vi "LD.vi"() -> ()   [LabVIEW 2022 SP3]
uses:
  <vilib>/Analysis/baseanly.llb/Mean (DBL).vi
  C:/Users/Public/OneDrive/Desktop/PMT program/SampleCodeLabView/Kinesis_with_LabVIEW_Examples_LV12 - v3/ThorLabs.MotionControl.KCube.DCServoCLI.dll
  PMT program/SampleCodeLabView/Kinesis_with_LabVIEW_Examples_LV12 - v3/ThorLabs.MotionControl.KCube.DCServoCLI.dll
  <vilib>/Utility/file.llb/Write Delimited Spreadsheet (string).vi
  <vilib>/Utility/file.llb/Write Delimited Spreadsheet (DBL).vi
  C:/Users/Public/OneDrive/Desktop/PMT program/SampleCodeLabView/Kinesis_with_LabVIEW_Examples_LV12 - v3/Thorlabs.MotionControl.Controls.dll
  PMT program/SampleCodeLabView/Kinesis_with_LabVIEW_Examples_LV12 - v3/Thorlabs.MotionControl.Controls.dll
  <vilib>/Analysis/NI_AALBase.lvlib
panel:
  in  "Waiting Time for motor":dbl=1500.0
  in  "OE1022D":refnum<visa-resource-name>
  in  "Total Steps":i32
  out "R Phase (B)":dbl[](graph)
  out "R (B)":dbl[](graph)
  out "R Phase (A)":dbl[](graph)
  out "R (A)":dbl[](graph)
  out "AUX-ADC4 (V)":sgl format="%.3f"
  out "AUX-ADC3 (V)":sgl format="%.3f"
  out "AUX-ADC1 (V)":sgl format="%.3f"
  out "AUX-ADC2 (V)":sgl format="%.3f"
  out "R":sgl caption="R (Vrms)" format="%.3p"
  out "X":sgl caption="X (Vrms)" format="%.3p"
  out "Y":sgl caption="Y (Vrms)" format="%.3p"
  out "θ (°)":sgl caption="θ (deg)" format="%.2f"
  out "频率 (Hz)":sgl caption="Freq (Hz)" format="%#.3f"
  out "噪声":sgl caption="Noise(Vrms)" format="%.3p"
  out "Rh1":sgl caption="Rh1 (Vrms)" format="%.3p"
  out "θh1 (°)":sgl caption="θh1 (deg)" format="%.2f"
  out "Rh2":sgl caption="Rh2 (Vrms)" format="%.3p"
  out "Xh2":sgl caption="Xh2 (Vrms)" format="%.3p"
  out "Yh2":sgl caption="Yh2 (Vrms)" format="%.3p"
  out "θh2 (°)":sgl caption="θh2 (deg)" format="%.2f"
  out "Xh1":sgl caption="Xh1 (Vrms)" format="%.3p"
  out "Yh1":sgl caption="Yh1 (Vrms)" format="%.3p"
  out "X 2":sgl caption="X (Vrms)" format="%.3p"
  out "θh2 (°) 2":sgl caption="θh2 (deg)" format="%.2f"
  out "Y 2":sgl caption="Y (Vrms)" format="%.3p"
  out "R 2":sgl caption="R (Vrms)" format="%.3p"
  out "θ (°) 2":sgl caption="θ (deg)" format="%.2f"
  out "频率 (Hz) 2":sgl caption="Freq (Hz)" format="%#.3f"
  out "噪声 2":sgl caption="Noise(Vrms)" format="%.3p"
  out "Rh2 2":sgl caption="Rh2 (Vrms)" format="%.3p"
  out "Yh2 2":sgl caption="Yh2 (Vrms)" format="%.3p"
  out "Xh2 2":sgl caption="Xh2 (Vrms)" format="%.3p"
  out "Xh1 2":sgl caption="Xh1 (Vrms)" format="%.3p"
  out "Yh1 2":sgl caption="Yh1 (Vrms)" format="%.3p"
  out "Rh1 2":sgl caption="Rh1 (Vrms)" format="%.3p"
  out "θh1 (°) 2":sgl caption="θh1 (deg)" format="%.2f"
  in  "file path (dialog if empty) 2":path=path "D:/LabData/Fan Fei/223.txt"
  in  "Lock  in Average Time":i32=500
  in  "Start":dbl
  out "Current Position":dbl
  in  "stepSize":dbl
  in  "direction":i32(ring)=1 items=["Forward"=1, "Backward"=2]
  in  "Motor Controller\nSerialNumber":string="27261255"
  in  "KCubeDCServoControl":refnum<k24>(container)
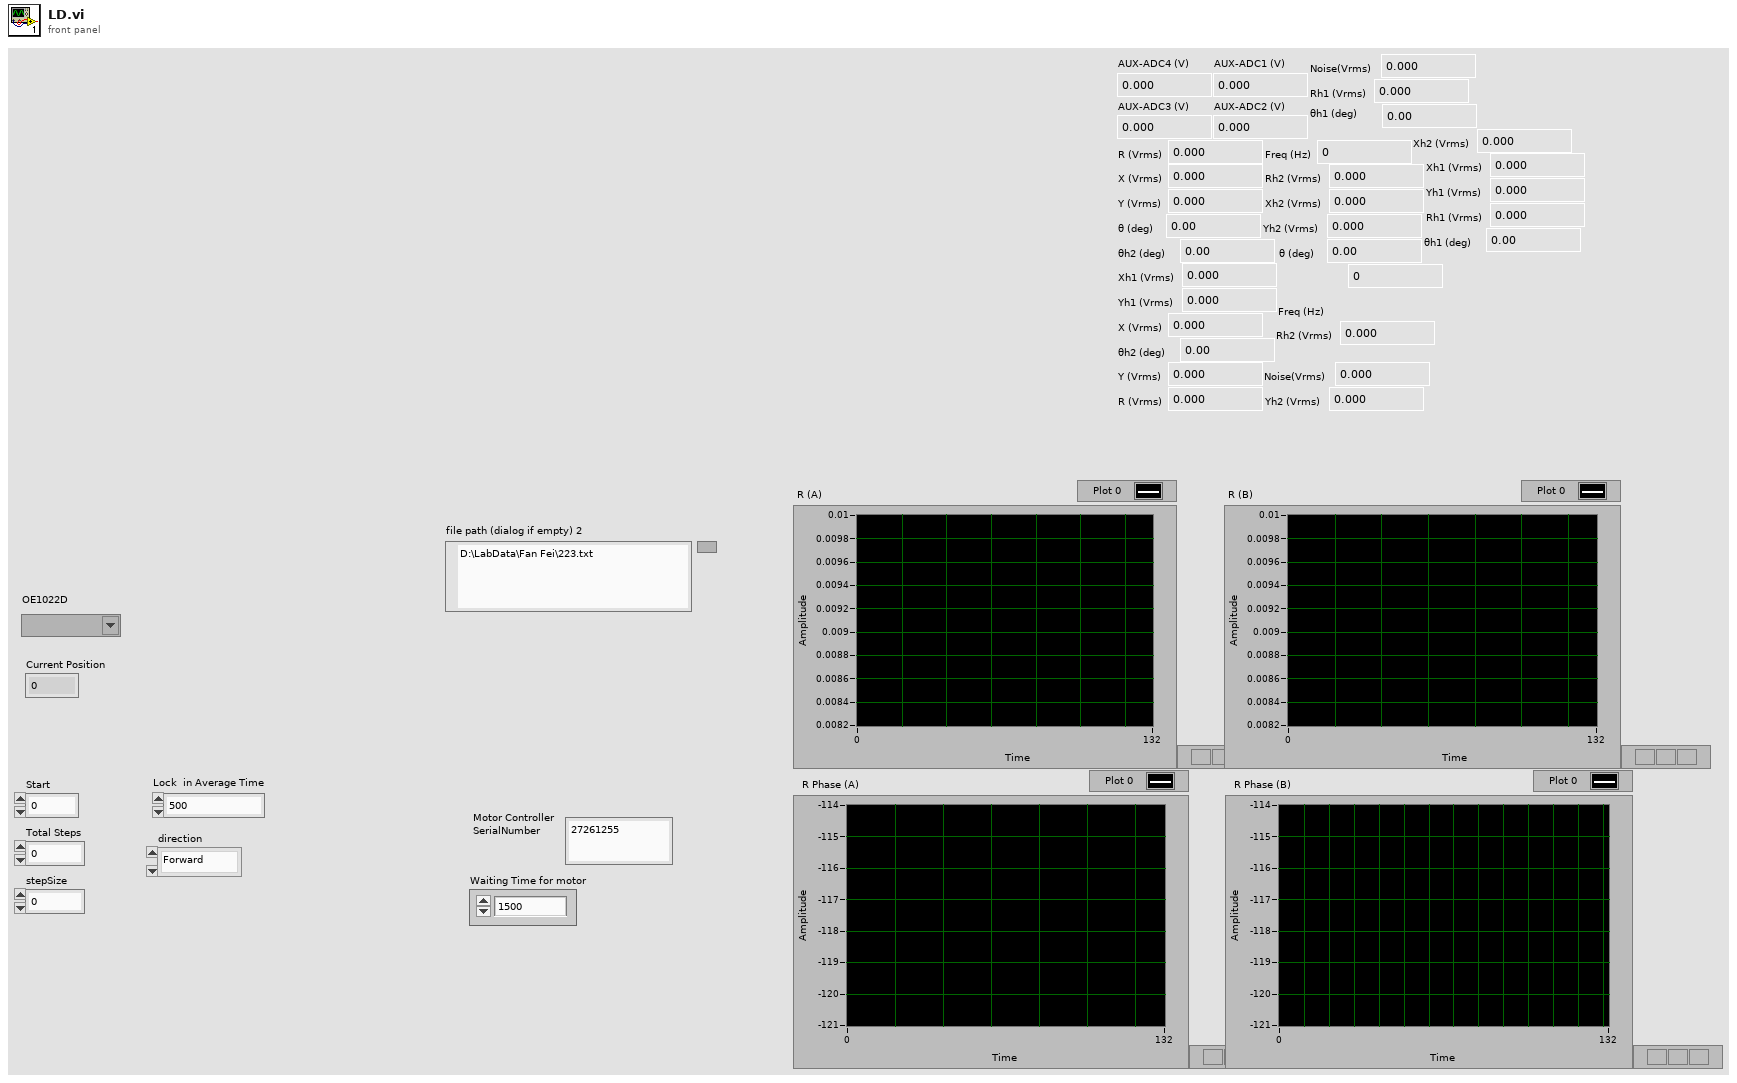
[diagram p1: front panel]
types:
  T1 = cluster{"AD1":dbl[], "AD2":dbl[], "AD3":dbl[], "AD4":dbl[]}
  T2 = cluster{"XB":dbl[], "YB":dbl[], "FrequencyB":dbl[], "NoiseB":dbl[], "Xh1B":dbl[], "Yh1B":dbl[], "Xh2B":dbl[], "Yh2B":dbl[], "Xh2B":dbl[]}
  T3 = cluster{"XA":dbl[], "YA":dbl[], "FrequencyA":dbl[], "NoiseA":dbl[], "Xh1A":dbl[], "Yh1A":dbl[], "Xh2A":dbl[], "Yh2A":dbl[]}
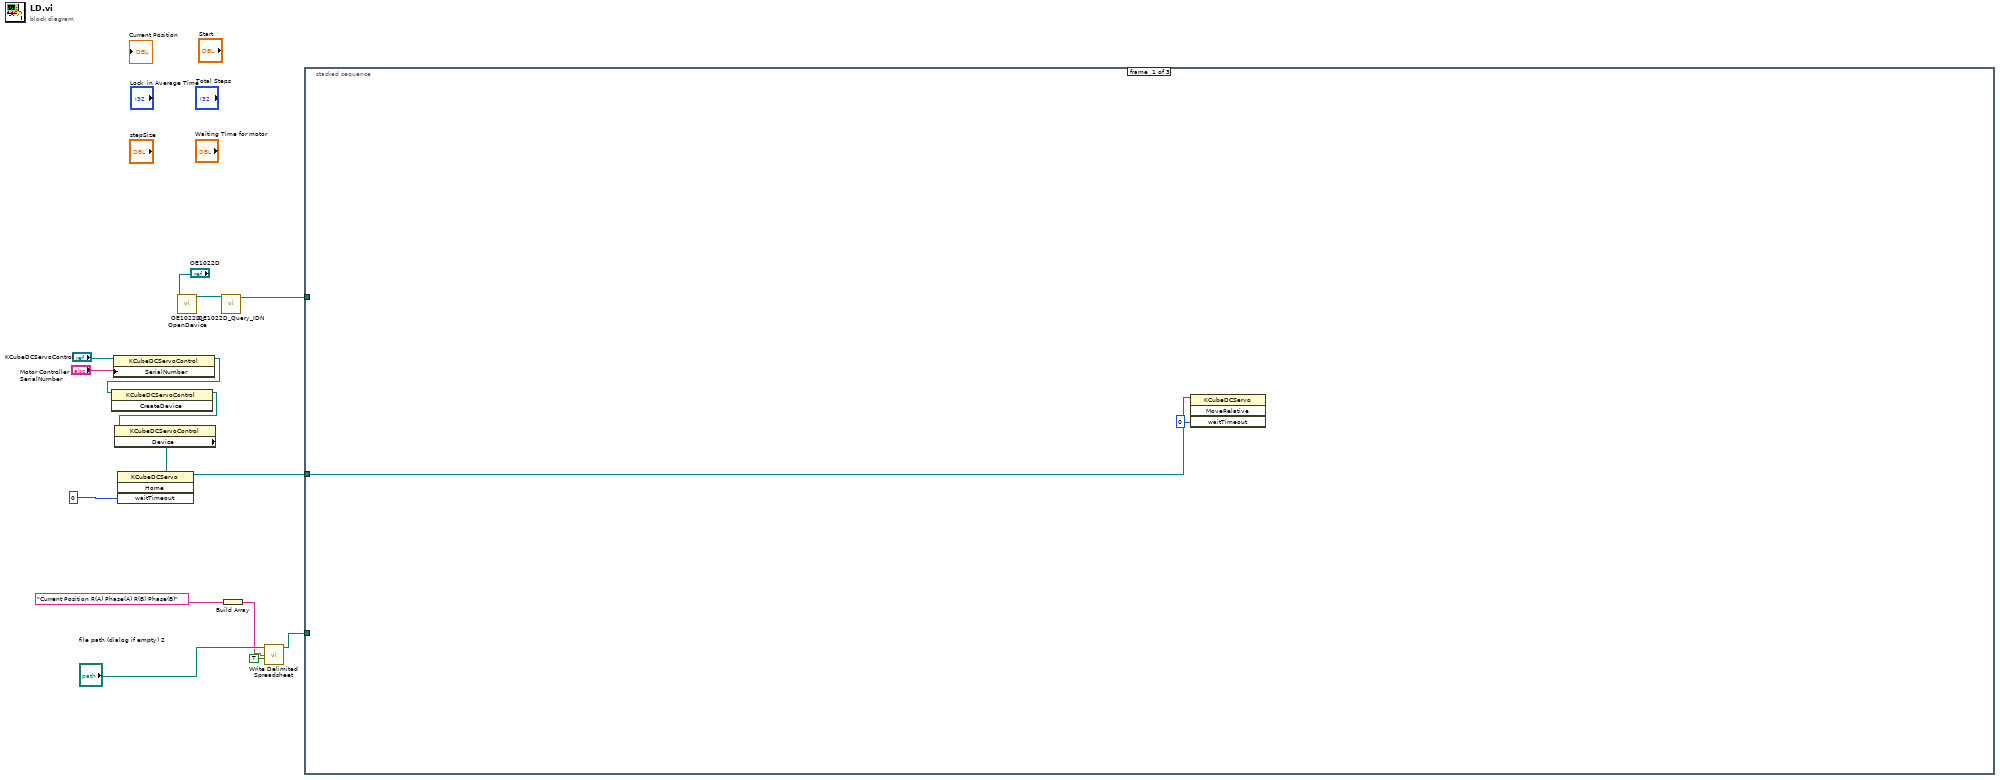
[diagram p0: block diagram]
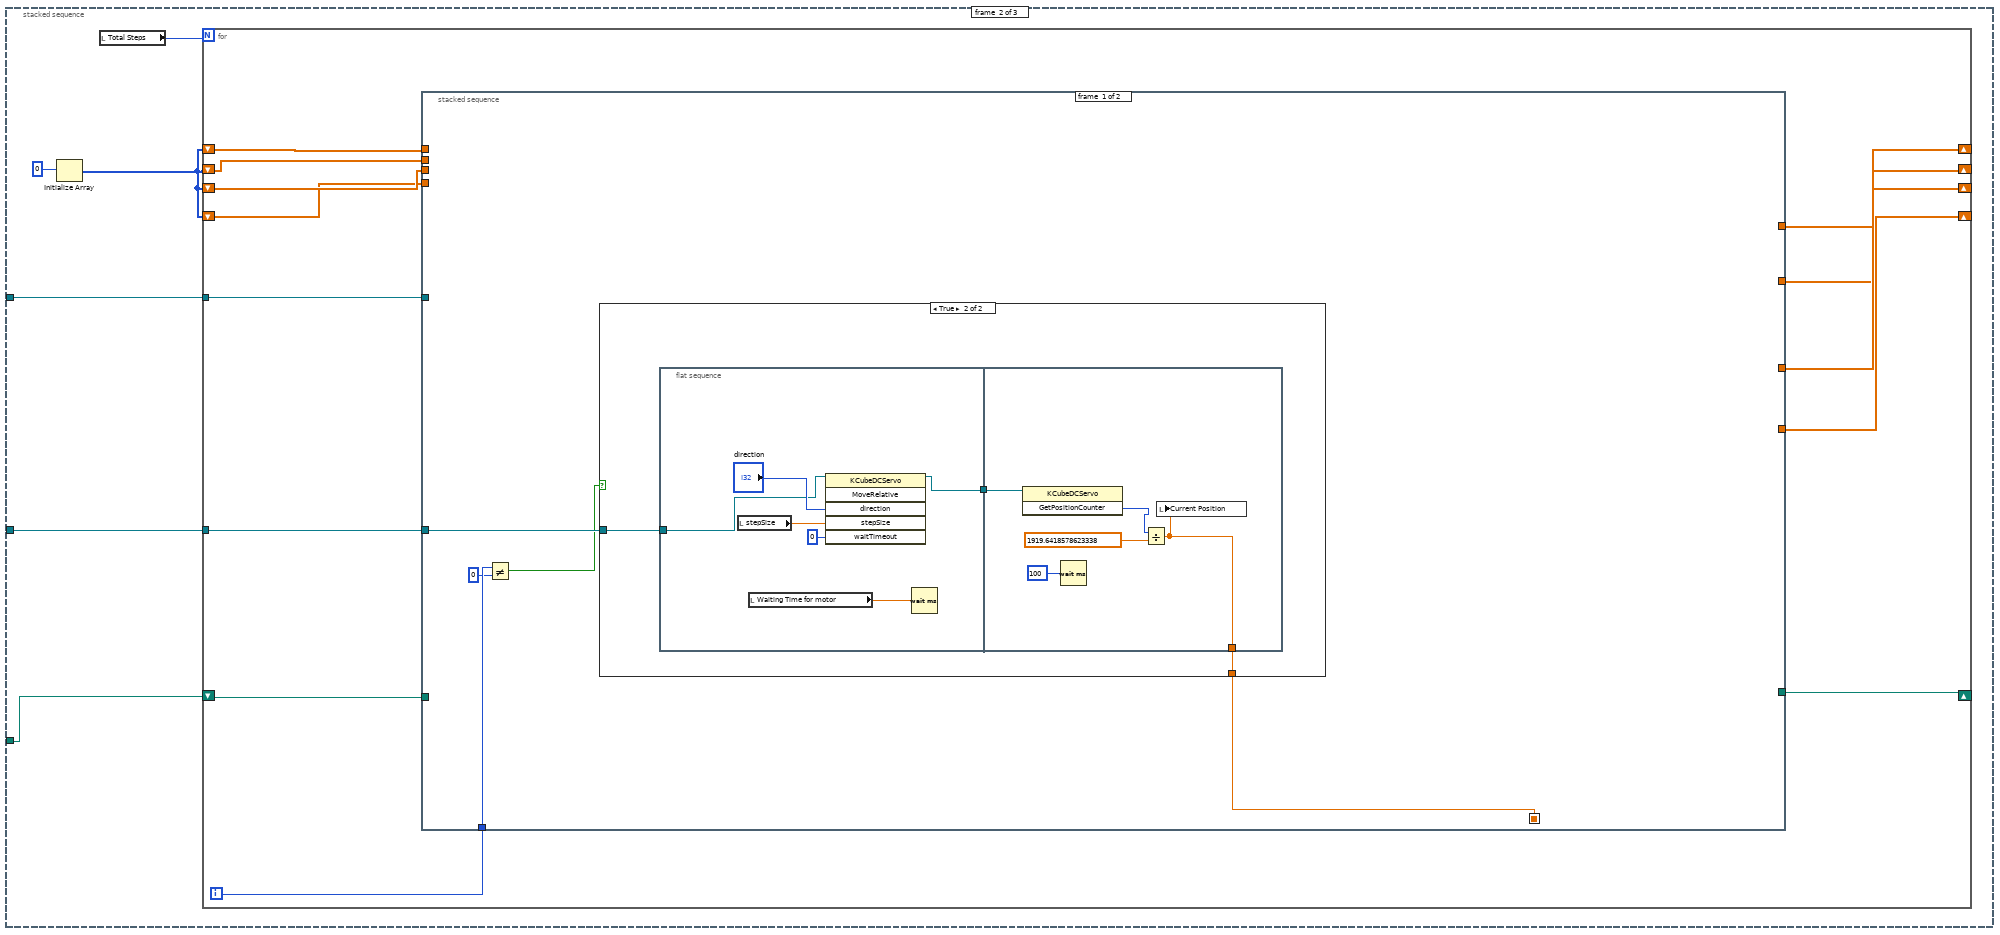
[diagram p2: hidden frame]
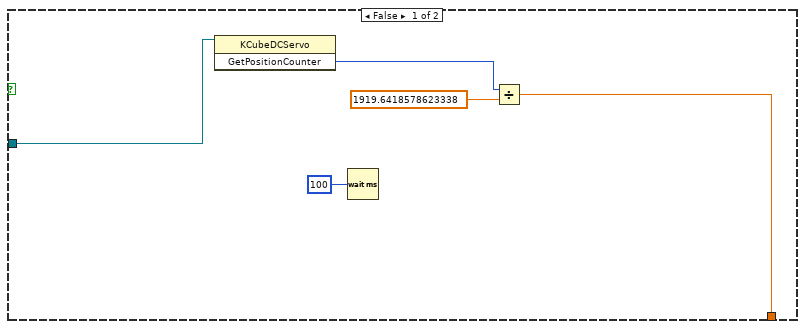
[diagram p3: hidden frame]
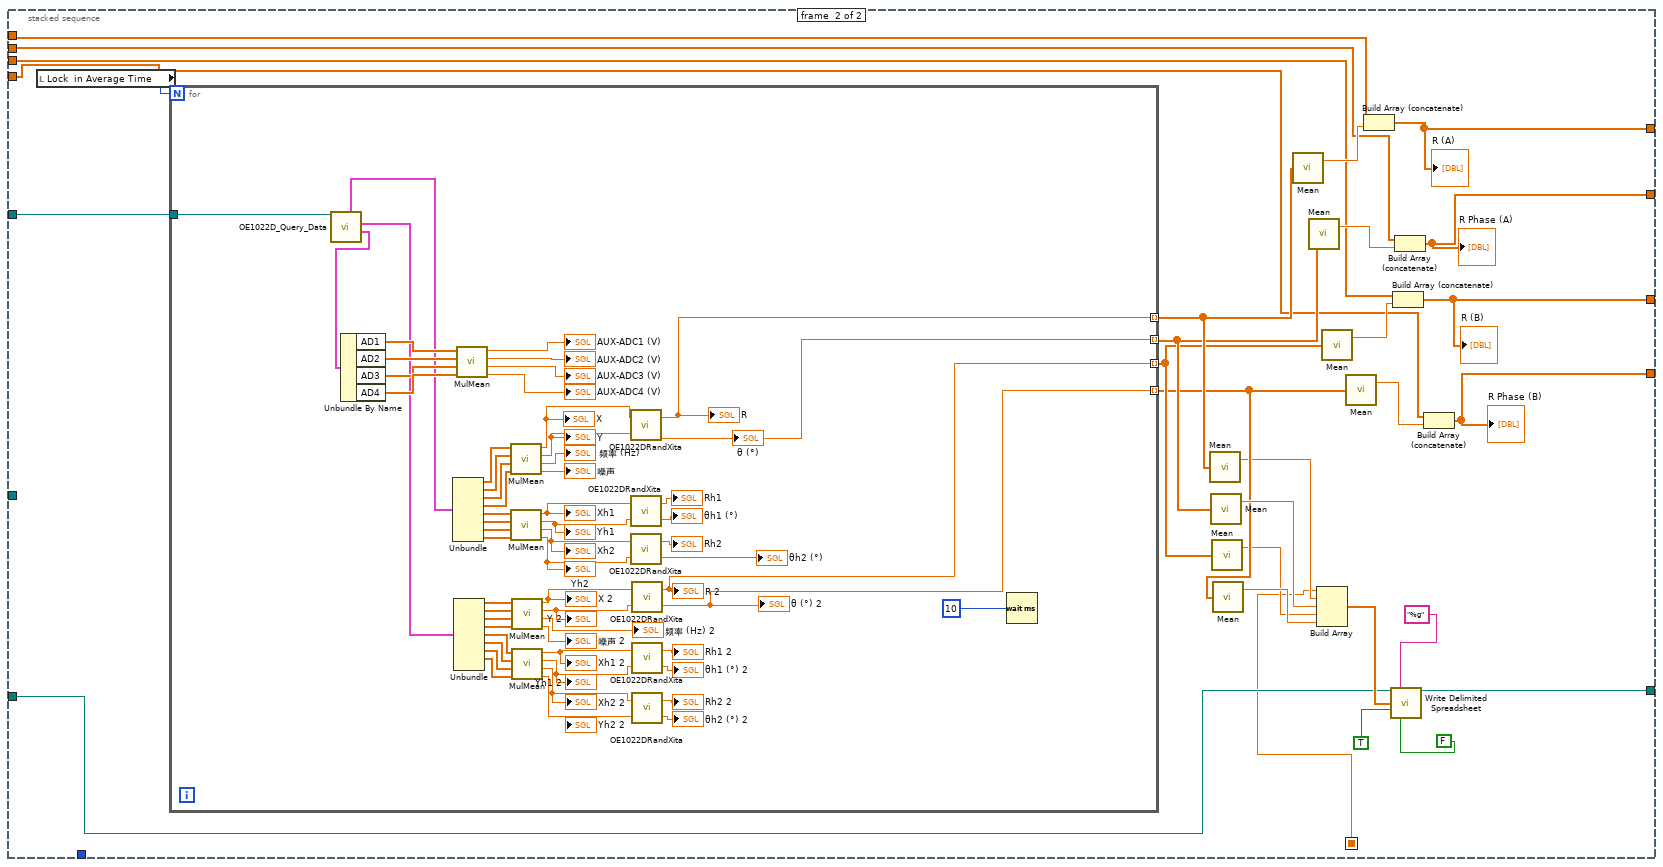
[diagram p4: hidden frame]
diagram:
  n1 = property class="KCubeDCServoControl"(reference="KCubeDCServoControl", "SerialNumber"="Motor Controller\nSerialNumber") -> (reference out=w14:refnum<k24>)  [unwired: 1 in, 1 out]
  n2 = invoke class="KCubeDCServoControl" method="CreateDevice"(reference=w14) -> (reference out=w10:refnum<k24>)  [unwired: 2 in, 2 out]
  n3 = property class="KCubeDCServoControl"(reference=w10) -> ("Device"=w11:refnum<k24>)  [unwired: 1 in, 2 out]
  n4 = invoke class="KCubeDCServo" method="Home"(reference=w11, "waitTimeout"=0) -> (reference out=w9:refnum<k24>)  [unwired: 2 in, 3 out]
  n5 = call "OE1022D_OpenDevice.vi"("VISA resource name"="OE1022D") -> ("VISA资源名称输出"=w2:refnum<visa-resource-name>)  [unwired: 17 in, 1 out]
  n6 = call "OE1022D_Query_IDN.vi"("VISA resource name"=w2) -> ("VISA resource name out"=w1:refnum<visa-resource-name>)  [unwired: 2 in, 2 out]
  n7 = Build Array("Current Position R(A) Phase(A) R(B) Phase(B)") -> (w6:string[])
  n8 = call-poly <vilib>:"Write Delimited Spreadsheet.vi"("file path (dialog if empty)"="file path (dialog if empty) 2", "1D data"=w6, "append to file? (new file:F)"=TRUE) -> ("new file path (Not A Path if cancelled)"=w4:path)  [unwired: 11 in, 1 out]
  n9 = stacked-sequence {
    tunnel: w9 -> [w17 w23 _]
    tunnel: w4 -> [_ w21 _]
    tunnel: w1 -> [_ w18 _]
    frame #0 {
      n10 = invoke class="KCubeDCServo" method="MoveRelative"(reference=w17, "waitTimeout"=0) -> ()  [unwired: 2 in, 4 out]
    }
    frame #1 {
      n11 = Initialize Array(0) -> (w19:i32[])  [unwired: 1 in]
      n12 = local read "Total Steps"() -> (w22:i32)
      n13 = for {
        N: w22 -> [_]
        tunnel: w23 -> [w36]
        shift-right: [w35] -> _
        shift-left: w21 -> [w34]
        shift-right: [w33] -> _
        shift-left: w19 -> [w29]
        shift-right: [w31] -> _
        shift-left: w19 -> [w28]
        shift-right: [w32] -> _
        shift-left: w19 -> [w27]
        shift-right: [w30] -> _
        shift-left: w19 -> [w26]
        tunnel: w18 -> [w25]
        i -> [w24]
        n14 = stacked-sequence {
          seq-local: [w37 _] -> [_ w62]
          tunnel: w36 -> [w41 _]
          tunnel: [_ w72] -> w35
          tunnel: w34 -> [_ w71]
          tunnel: [_ w70] -> w33
          tunnel: [_ w69] -> w32
          tunnel: [_ w68] -> w31
          tunnel: [_ w67] -> w30
          tunnel: w29 -> [_ w66]
          tunnel: w28 -> [_ w65]
          tunnel: w27 -> [_ w64]
          tunnel: w26 -> [_ w63]
          tunnel: w25 -> [_ w61]
          tunnel: w24 -> [w40 _]
          frame #0 {
            n15 = Not Equal?(x=w40, y=0) -> (x != y?=w38:bool)
            n16 = case shown="True" w38 {
              tunnel: w41 -> [w46 w47]
              tunnel: [w43 w48] -> w37
              frame False {
                n17 = invoke class="KCubeDCServo" method="GetPositionCounter"(reference=w46) -> ("GetPositionCounter"=w44:i32)  [unwired: 2 in, 2 out]
                n18 = Wait (ms)(milliseconds to wait=100) -> ()  [unwired: 1 out]
                n19 = Divide(x=w44, y=1919.6418578623338) -> (x/y=w43:dbl)
              }
              frame True {
                n20 = flat-sequence {
                  tunnel: [w53] -> w49
                  tunnel: w47 -> [w50]
                  tunnel: w49 -> [w58]
                  tunnel: [w56] -> w48
                  frame #0 {
                    n21 = local read "stepSize"() -> (w52:dbl)
                    n22 = local read "Waiting Time for motor"() -> (w51:dbl)
                    n23 = invoke class="KCubeDCServo" method="MoveRelative"(reference=w50, "direction"="direction", "stepSize"=w52, "waitTimeout"=0) -> (reference out=w53:refnum<k24>)  [unwired: 2 in, 5 out]
                    n24 = Wait (ms)(milliseconds to wait=w51) -> ()  [unwired: 1 out]
                  }
                  frame #1 {
                    n25 = invoke class="KCubeDCServo" method="GetPositionCounter"(reference=w58) -> ("GetPositionCounter"=w60:i32)  [unwired: 2 in, 2 out]
                    n26 = Wait (ms)(milliseconds to wait=100) -> ()  [unwired: 1 out]
                    n27 = Divide(x=w60, y=1919.6418578623338) -> (x/y=w56:dbl)
                    n28 = local write "Current Position"(w56) -> ()
                  }
                }
              }
            }
          }
          frame #1 {
            n29 = local read "Lock  in Average Time"() -> (w73:i32)
            n30 = for {
              N: w73 -> [_]
              tunnel: [w94] -> w80 mode=indexing
              tunnel: [w93] -> w79 mode=indexing
              tunnel: [w92] -> w78 mode=indexing
              tunnel: [w91] -> w77 mode=indexing
              tunnel: w61 -> [w90]
              n31 = call "OE1022D_Query_Data.vi"("VISA resource name"=w90) -> ("输出簇ADC"=w95:T1, "输出簇B"=w97:T2, "输出簇A"=w96:T3)  [unwired: 4 in, 2 out]
              n32 = Unbundle By Name(w95) -> ("AD1"=w143:dbl[], "AD2"=w144:dbl[], "AD3"=w145:dbl[], "AD4"=w146:dbl[])
              n33 = Unbundle(w96) -> ("XA"=w107:dbl[], "YA"=w108:dbl[], "FrequencyA"=w109:dbl[], "NoiseA"=w110:dbl[], "Xh1A"=w115:dbl[], "Yh1A"=w116:dbl[], "Xh2A"=w117:dbl[], "Yh2A"=w118:dbl[])
              n34 = Unbundle(w97) -> ("XB"=w132:dbl[], "YB"=w131:dbl[], "FrequencyB"=w130:dbl[], "NoiseB"=w129:dbl[], "Xh1B"=w128:dbl[], "Yh1B"=w127:dbl[], "Xh2B"=w126:dbl[], "Yh2B"=w125:dbl[])  [unwired: 1 out]
              n35 = call "MulMean.vi"("IN 4"=w146, "IN 3"=w145, "IN 2"=w144, "IN 1"=w143) -> ("mean 4"=→"AUX-ADC4 (V)":dbl, "mean 3"=→"AUX-ADC3 (V)":dbl, "mean 2"=→"AUX-ADC2 (V)":dbl, "mean 1"=→"AUX-ADC1 (V)":dbl)  [unwired: 4 in]
              n36 = call "MulMean.vi"("IN 4"=w110, "IN 3"=w109, "IN 2"=w108, "IN 1"=w107) -> ("mean 4"=→"噪声":dbl, "mean 3"=→"频率 (Hz)":dbl, "mean 2"=w113:dbl, "mean 1"=w112:dbl)  [unwired: 4 in]
              "X" <- w112
              "Y" <- w113
              n37 = call "MulMean.vi"("IN 4"=w118, "IN 3"=w117, "IN 2"=w116, "IN 1"=w115) -> ("mean 4"=w122:dbl, "mean 3"=w121:dbl, "mean 2"=w120:dbl, "mean 1"=w119:dbl)  [unwired: 4 in]
              "Xh2" <- w121
              "Yh2" <- w122
              "Xh1" <- w119
              "Yh1" <- w120
              n38 = call "MulMean.vi"("IN 4"=w129, "IN 3"=w130, "IN 2"=w131, "IN 1"=w132) -> ("mean 4"=→"噪声 2":dbl, "mean 3"=→"频率 (Hz) 2":dbl, "mean 2"=w136:dbl, "mean 1"=w135:dbl)  [unwired: 4 in]
              "X 2" <- w135
              "Y 2" <- w136
              n39 = call "MulMean.vi"("IN 4"=w125, "IN 3"=w126, "IN 2"=w127, "IN 1"=w128) -> ("mean 4"=w140:dbl, "mean 3"=w139:dbl, "mean 2"=w138:dbl, "mean 1"=w137:dbl)  [unwired: 4 in]
              "Xh2 2" <- w139
              "Xh1 2" <- w137
              "Yh1 2" <- w138
              n40 = call "OE1022DRandXita.vi"("Y"=w113, "X"=w112) -> ("θ (°)"=w93:dbl, "R"=w94:dbl)
              "R" <- w94
              "θ (°)" <- w93
              n41 = call "OE1022DRandXita.vi"("Y"=w120, "X"=w119) -> ("θ (°)"=→"θh1 (°)":dbl, "R"=→"Rh1":dbl)
              n42 = call "OE1022DRandXita.vi"("Y"=w122, "X"=w121) -> ("θ (°)"=→"θh2 (°)":dbl, "R"=→"Rh2":dbl)
              n43 = call "OE1022DRandXita.vi"("Y"=w136, "X"=w135) -> ("θ (°)"=w91:dbl, "R"=w92:dbl)
              "R 2" <- w92
              "θ (°) 2" <- w91
              n44 = call "OE1022DRandXita.vi"("Y"=w138, "X"=w137) -> ("θ (°)"=→"θh1 (°) 2":dbl, "R"=→"Rh1 2":dbl)
              n45 = call "OE1022DRandXita.vi"("Y"=w140, "X"=w139) -> ("θ (°)"=→"θh2 (°) 2":dbl, "R"=→"Rh2 2":dbl)
              n46 = Wait (ms)(milliseconds to wait=10) -> ()  [unwired: 1 out]
            }
            n47 = call-poly <vilib>:"Mean.vi"("X"=w80) -> ("mean"=w74:dbl)  [unwired: 1 out]
            n48 = call-poly <vilib>:"Mean.vi"("X"=w79) -> ("mean"=w86:dbl)  [unwired: 1 out]
            n49 = call-poly <vilib>:"Mean.vi"("X"=w78) -> ("mean"=w75:dbl)  [unwired: 1 out]
            n50 = call-poly <vilib>:"Mean.vi"("X"=w77) -> ("mean"=w76:dbl)  [unwired: 1 out]
            n51 = call-poly <vilib>:"Mean.vi"("X"=w80) -> ("mean"=w83:dbl)  [unwired: 1 out]
            n52 = call-poly <vilib>:"Mean.vi"("X"=w79) -> ("mean"=w84:dbl)  [unwired: 1 out]
            n53 = Build Array(w62, w74, w86, w75, w76) -> (w85:dbl[])
            n54 = call-poly <vilib>:"Mean.vi"("X"=w78) -> ("mean"=w82:dbl)  [unwired: 1 out]
            n55 = call-poly <vilib>:"Mean.vi"("X"=w77) -> ("mean"=w81:dbl)  [unwired: 1 out]
            n56 = Build Array (concatenate)(w66, w83) -> (w70:dbl[])
            "R (A)" <- w70
            n57 = call-poly <vilib>:"Write Delimited Spreadsheet.vi"("file path (dialog if empty)"=w71, "format (%.3f)"="%g", "1D data"=w85, "append to file? (new file:F)"=TRUE, "transpose? (no:F)"=FALSE) -> ("new file path (Not A Path if cancelled)"=w72:path)  [unwired: 9 in, 1 out]
            n58 = Build Array (concatenate)(w64, w82) -> (w69:dbl[])
            "R (B)" <- w69
            n59 = Build Array (concatenate)(w65, w84) -> (w68:dbl[])
            "R Phase (A)" <- w68
            n60 = Build Array (concatenate)(w63, w81) -> (w67:dbl[])
            "R Phase (B)" <- w67
          }
        }
      }
    }
    frame #2 {
    }
  }
